vi "Write Display Function.vi"(8 "error in (no error)":errorcluster, 9 "Display Function":T1, 10 "Session In":refnum<class "Session.lvclass">, 11 "PCF8574 I2C LCD in":refnum<class "PCF8574 I2C LCD.lvclass">) -> (0 "error out":errorcluster, 2 "Session Out":refnum<class "Session.lvclass">, 3 "PCF8574 I2C LCD out":refnum<class "PCF8574 I2C LCD.lvclass">)   [LabVIEW 2020, in "CTI-Peripheral.lvlib" / "PCF8574 I2C LCD.lvclass"]
uses:
  PCF8574 I2C LCD.lvclass
  CTI/Session/Session.lvclass
  HD44780 LCD/Display Function.ctl
  Character LCD/Bus Mode.ctl
  Character LCD/Lines.ctl
  Character LCD/Glyph Size.ctl
  HD44780 LCD/Command.ctl
  PCF8574 I2C LCD.lvclass/PCF8574 I2C LCD.ctl
  HD44780 LCD/HD44780 LCD.lvlib
  Character LCD/Char LCD.lvclass
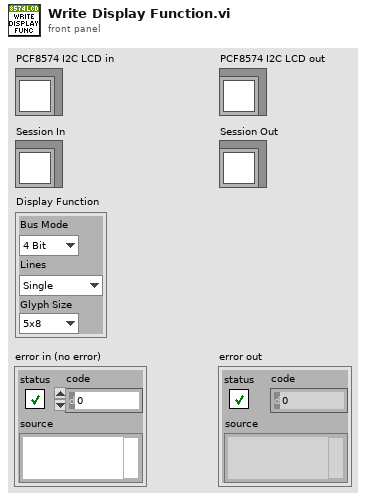
[diagram p1: front panel]
types:
  T1 = typedef "CTI-Peripheral.lvlib/HD44780 LCD.lvlib/Display Function.ctl" = cluster{"Bus Mode":T2, "Lines":T3, "Glyph Size":T4}
  T2 = typedef "CTI-Peripheral.lvlib/Char LCD.lvclass/Bus Mode.ctl" = enum8{"4 Bit", "8 Bit"}
  T3 = typedef "CTI-Peripheral.lvlib/Char LCD.lvclass/Lines.ctl" = enum8{"Single", "Multiline"}
  T4 = typedef "CTI-Peripheral.lvlib/Char LCD.lvclass/Glyph Size.ctl" = enum8{"5x8", "5x10"}
  T5 = typedef "CTI-Peripheral.lvlib/HD44780 LCD.lvlib/Command.ctl" = enum16{"ClearDisplay", "ReturnHome", "EntryModeSet", "DisplayControl", "CursorShift", "FunctionSet", "SetCGRamAddr", "SetDDRamAddr"}
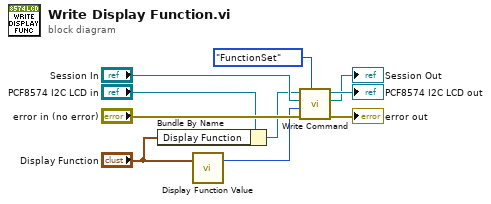
[diagram p0: block diagram]
diagram:
  n1 = Bundle By Name(cluster="PCF8574 I2C LCD in", "Display Function"="Display Function") -> (w3:refnum<class "PCF8574 I2C LCD.lvclass">)
  n2 = call "Display Function Value.vi"("Display Function"="Display Function") -> ("DisplayFunc"=w1:u8)  [unwired: 6 in]
  n3 = call "Write Command.vi"("Command"=Command."FunctionSet", "error in (no error)"="error in (no error)", "Value"=w1, "Session In"="Session In", "PCF8574 I2C LCD in"=w3) -> ("error out"=→"error out":errorcluster, "Session Out"=→"Session Out":refnum<class "Session.lvclass">, "PCF8574 I2C LCD out"=→"PCF8574 I2C LCD out":refnum<class "PCF8574 I2C LCD.lvclass">)  [unwired: 4 in]
